vi "SetCellStyle.vi"(4 "Column":i32, 6 "Row":i32, 8 "error in (no error)":errorcluster, 10 "CellStyle.lvclass":refnum<class "CellStyle.lvclass">, 11 "DataGridView in":refnum<class "DataGridView.lvclass">) -> (0 "error out":errorcluster, 3 "DataGridView out":refnum<class "DataGridView.lvclass">)   [LabVIEW 2014, in "DataGridView.lvclass"]
uses:
  DataGridView.lvclass
  CellStyle/CellStyle.lvclass
  CellStyle/CellStyle.lvclass/CellStyle.ctl
  DataGridView.lvclass/DataGridView.ctl
  System.Windows.Forms
  CellStyle/Properties/Read cellStyle.vi
  Read DataGridView.vi
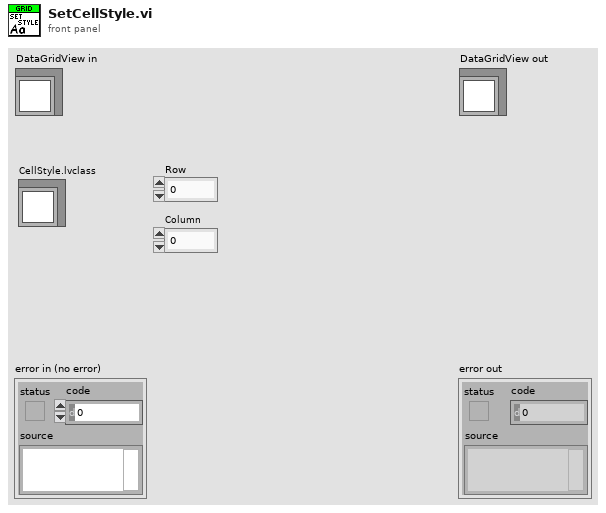
[diagram p1: front panel]
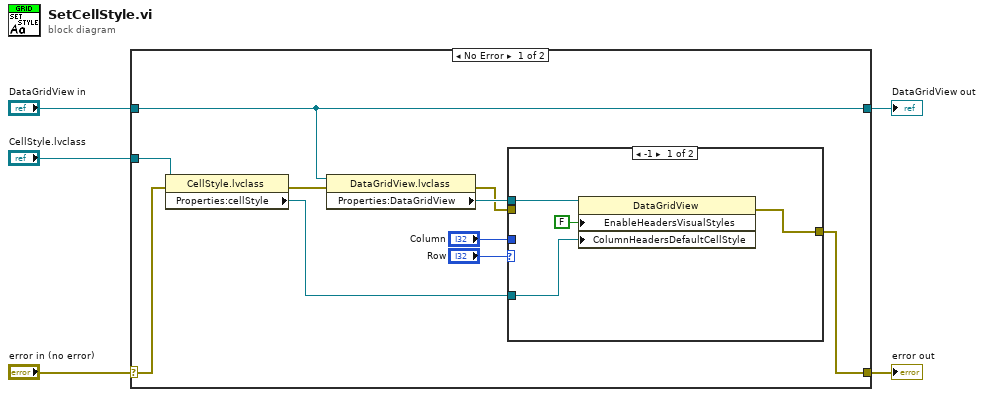
[diagram p0: block diagram]
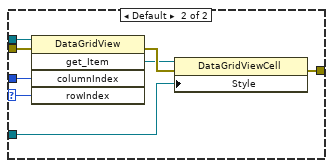
[diagram p2: hidden frame]
diagram:
  n1 = case shown="No Error" "error in (no error)" {
    selector: "error in (no error)" -> [w14 w29]
    tunnel: [w11 w29] -> w4
    tunnel: [w13 w28] -> w2
    tunnel: "DataGridView in" -> [w13 w28]
    tunnel: "CellStyle.lvclass" -> [w15 _]
    frame No Error {
      n2 = property class="CellStyle.lvclass"(reference=w15, error in=w14) -> (error out=w12:errorcluster, "Properties:cellStyle"=w7:refnum<k24>)  [unwired: 1 out]
      n3 = property class="DataGridView.lvclass"(reference=w13, error in=w12) -> (error out=w8:errorcluster, "Properties:DataGridView"=w10:refnum<k24>)  [unwired: 1 out]
      n4 = case shown="-1" "Row" {
        selector: "Row" -> [_ w20]
        tunnel: [w18 w27] -> w11
        tunnel: w10 -> [w19 w26]
        tunnel: "Column" -> [_ w25]
        tunnel: w8 -> [_ w24]
        tunnel: w7 -> [w17 w21]
        frame -1 {
          n5 = property class="DataGridView"(reference=w19, "EnableHeadersVisualStyles"=FALSE, "ColumnHeadersDefaultCellStyle"=w17) -> (error out=w18:errorcluster)  [unwired: 1 in, 1 out]
        }
        frame Default {
          n6 = invoke class="DataGridView" method="get_Item"(reference=w26, error in=w24, "columnIndex"=w25, "rowIndex"=w20) -> (error out=w23:errorcluster, "get_Item"=w22:refnum<k24>)  [unwired: 1 in, 3 out]
          n7 = property class="DataGridViewCell"(reference=w22, error in=w23, "Style"=w21) -> (error out=w27:errorcluster)  [unwired: 1 out]
        }
      }
    }
    frame Error {
    }
  }
  "error out" <- w4
  "DataGridView out" <- w2
